vi "Send Stop Event MessengerM.vi"(7 "subchannel":i32, 10 "sync in":errorcluster) -> (2 "channel":T1)   [LabVIEW 2019, in "Cmd-Data Event MessengerM Messages.lvlib"]
doc: "Sends a message with command STOP and empty Data Variant. This VI executes normally even if there is an error at sync in."
uses:
  Cmd-Data Event MessengerM Messages.lvlib
  <resource>/Channels/Event MessengerM/Event MessengerM.lvlib
  <resource>/Channels/Event MessengerM/))Channel.ctl
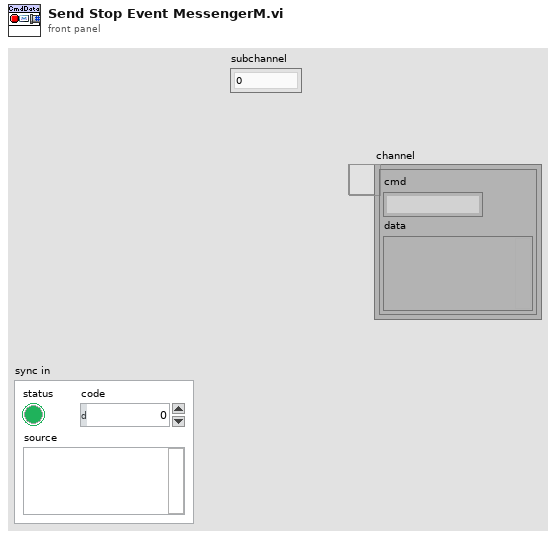
[diagram p1: front panel]
types:
  T1 = typedef "Event MessengerM.lvlib/))Channel.ctl" = refnum<queue>
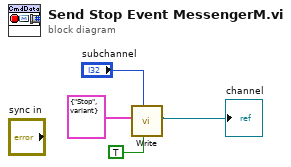
[diagram p0: block diagram]
diagram:
  n1 = call <resource>:"Write.vi"("high priority? (F)"=TRUE, "subchannel (0)"="subchannel", "element"=cluster{"cmd":string, "data":variant} {"cmd"="Stop", "data"=variant} ("message")) -> ("channel"=→"channel":T1)  [unwired: 7 in, 1 out]
